vi "CreateDataStructures.vi"(8 "Error In":errorcluster) -> (0 "Error Out":errorcluster, 3 "Data Structures":T1)   [LabVIEW 2013]
uses:
  DataStructures.ctl
  HardwareDisplayData.ctl
  HardwareLogData.ctl
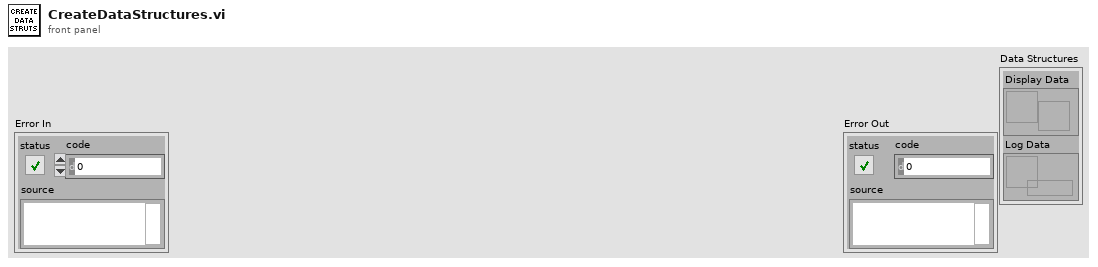
[diagram p1: front panel]
types:
  T1 = typedef "DataStructures.ctl" = cluster{"Display Data":refnum<notifier>, "Log Data":refnum<queue>}
  T2 = typedef "HardwareLogData.ctl" = cluster{"Timestamp":timestamp, "Data":T3}
  T3 = typedef "HardwareDisplayData.ctl" = cluster{"DUT Names":string[][], "SMU":dbl[][], "Port":bool[]}
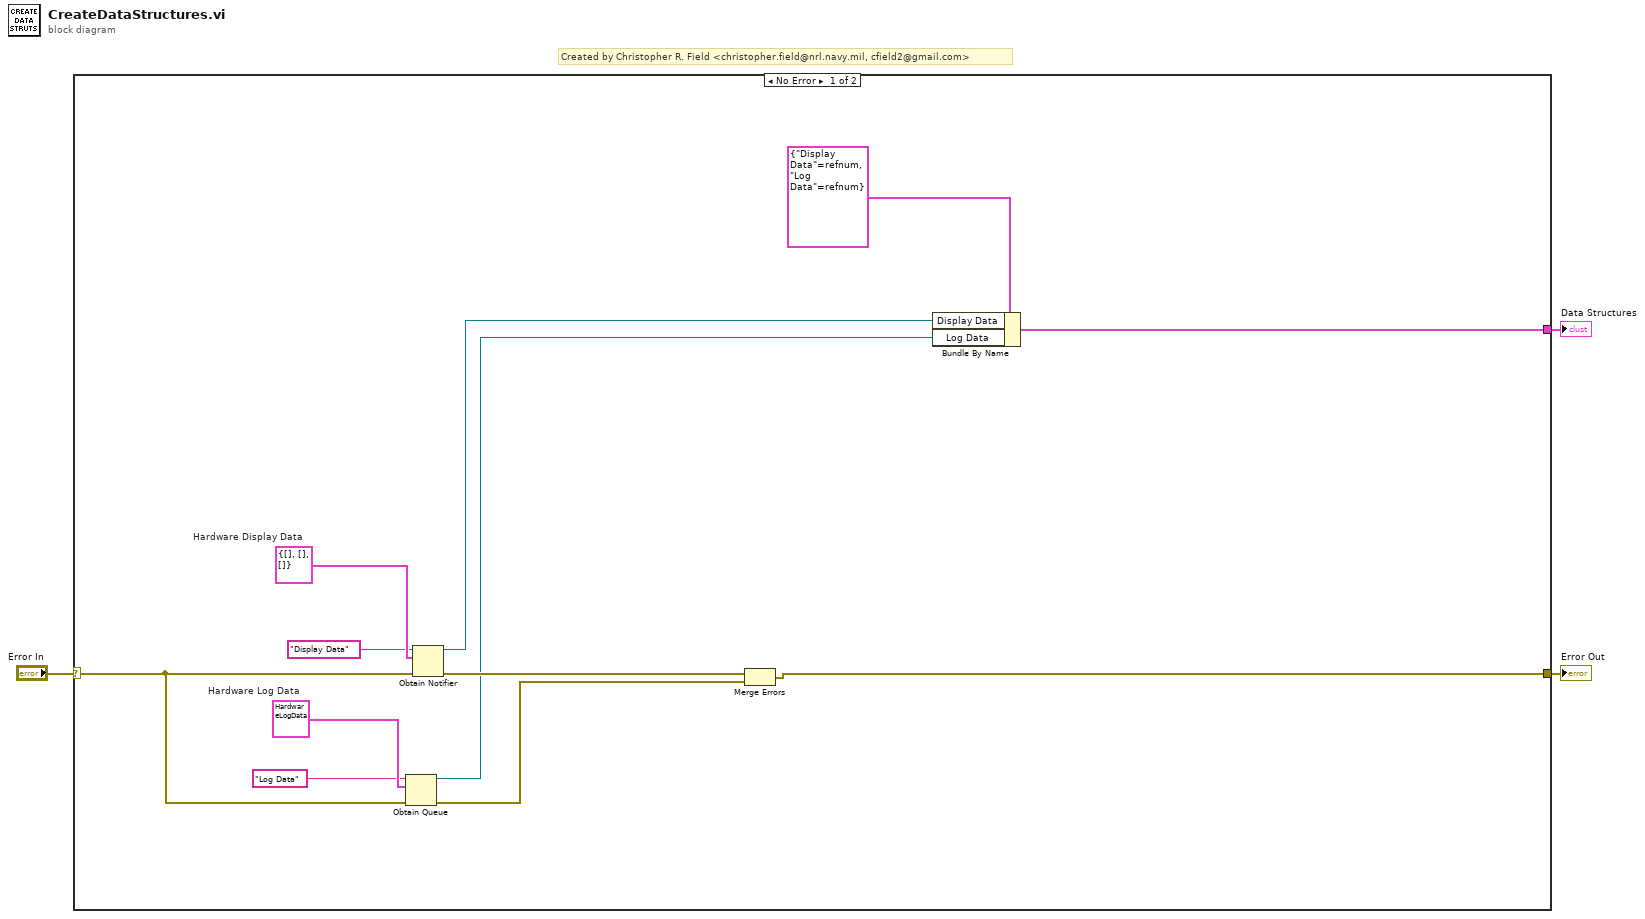
[diagram p0: block diagram]
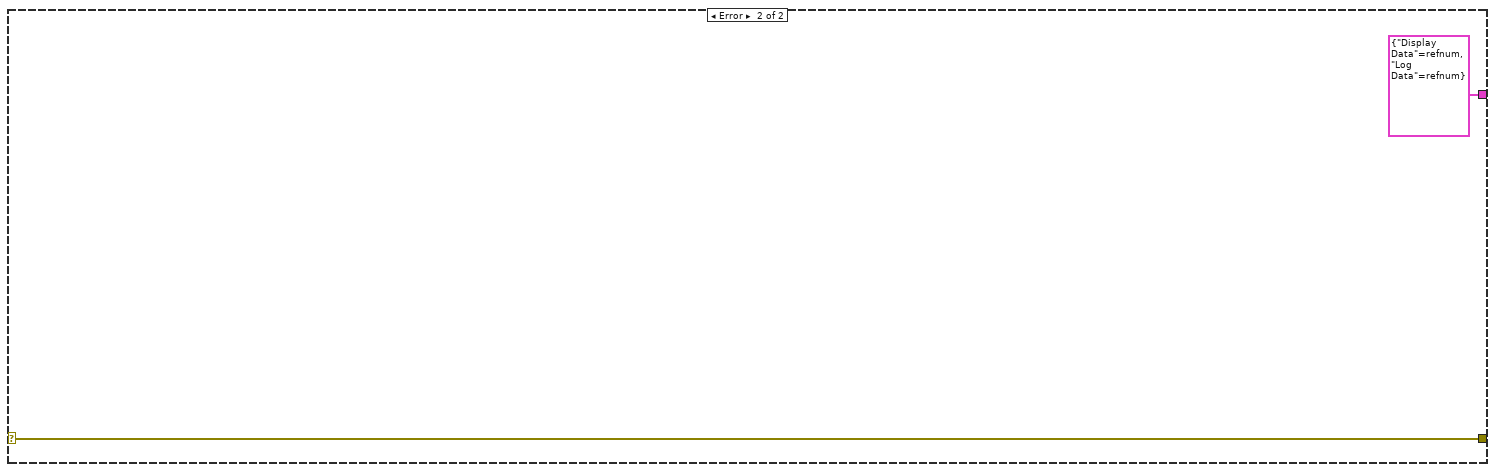
[diagram p2: hidden frame]
diagram:
  # "Created by Christopher R. Field <christopher.field@nrl.navy.mil, cfield2@gmail.com>"
  n1 = case shown="No Error" "Error In" {
    selector: "Error In" -> [w8 w17]
    tunnel: [w4 w17] -> w2
    tunnel: [w11 T1 {"Display Data"=refnum, "Log Data"=refnum} ("Data Structures")] -> w1
    frame No Error {
      w10 = T2 {"Timestamp"=timestamp(0 s since 1904-01-01), "Data"={"DUT Names"=[], "SMU"=[], "Port"=[]}}  # Hardware Log Data
      w15 = T3 {"DUT Names"=[], "SMU"=[], "Port"=[]}  # Hardware Display Data
      n2 = Obtain Queue(name (unnamed)="Log Data", element data type=w10, error in (no error)=w8) -> (queue out=w5:refnum<queue>, error out=w6:errorcluster)  [unwired: 2 in, 1 out]
      n3 = Obtain Notifier(name (unnamed)="Display Data", notification data type=w15, error in (no error)=w8) -> (notifier out=w12:refnum<notifier>, error out=w7:errorcluster)  [unwired: 1 in, 1 out]
      n4 = Merge Errors(w7, w6) -> (w4:errorcluster)
      n5 = Bundle By Name(cluster=T1 {"Display Data"=refnum, "Log Data"=refnum} ("Data Structures"), "Display Data"=w12, "Log Data"=w5) -> (w11:T1)
    }
    frame Error {
    }
  }
  "Error Out" <- w2
  "Data Structures" <- w1
